vi "test wydajnosci akzwizycji.vi"() -> ()   [LabVIEW 2014]
uses:
  Kontrolki/KartaDAQ/ACQ analog channel config new.ctl
  Kontrolki/KartaDAQ/ACQ counter channel config.ctl
  Kontrolki/KartaDAQ/ACQ Params.ctl
  Kontrolki/KartaDAQ/ACQ all read tasks.ctl
  Kontrolki/FVGs/FVG akcje podstawowa.ctl
panel:
  out "srednie przysp":dbl
  out "srednia predk":dbl
  in  "generuj plik":bool
  in  "file path":path
  in  "Tab Control":enum32{"Page 1", "Page 2"}(tab)
  out "Waveform Graph":waveform(dbl)[](graph)
  out "Waveform Graph 3":waveform(dbl)[](graph)
  out "deleted portion":dbl[](array[numeric]) format="%.8f"
  out "Array":T1(array[cluster])
  out "size(s)":i32
  out "wektor size(s)":i32
  in  "użyj x0":bool
  out "okno dt":dbl
  out "dt":dbl
  out "średnia delay":dbl
  out "delay":dbl format="%.2f"
  in  "stop":bool
  in  "Urządzenie":tag="Dev1"
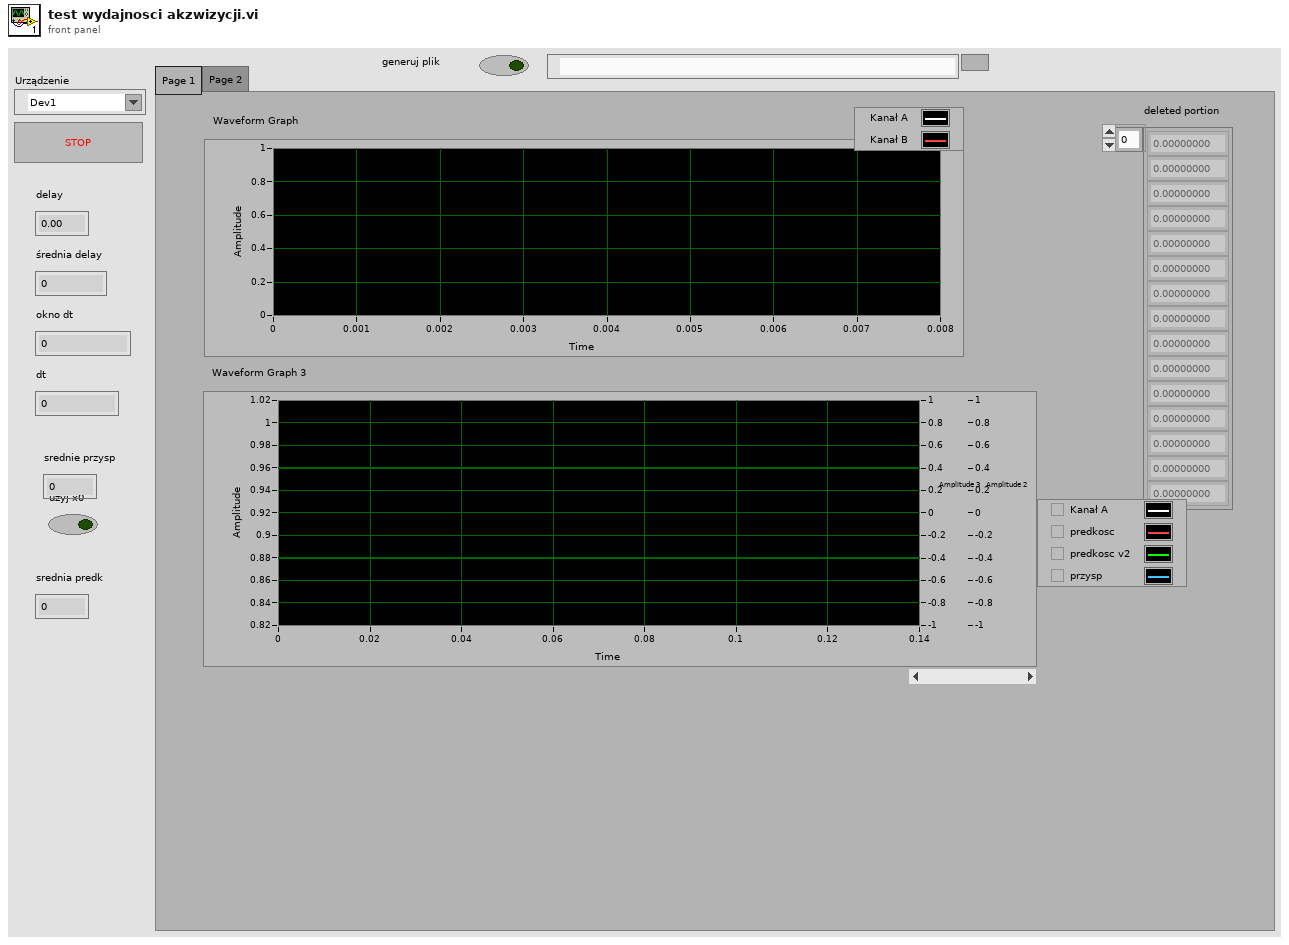
[diagram p1: front panel]
types:
  T1 = cluster{"dane":dbl[], "wygladzone":dbl[], "pochodna":dbl[], "pochodna wygl":dbl[]}[]
  T2 = typedef "ACQ all read tasks.ctl" = cluster{"Analog ref":refnum<k21>, "Enkoder X ref":refnum<k21>, "Enkoder Y ref":refnum<k21>, "Generator ref":refnum<k21>}
  T3 = typedef "ACQ Params.ctl" = cluster{"Analog":cluster{"minimum value":dbl, "maximum value":dbl}, "Digital":cluster{"minimum value":dbl, "maximum value":dbl}, "Time":cluster{"sample mode":i32, "samples per channel in":i32, "rate":dbl, "active edge":i32}, "AI common":cluster{"input terminal configuration":i32, "source":string}, "Enkoder":cluster{"channel1 name":string, "channel2 name":string, "units":i32, "initial position":dbl, "distance per pulse":dbl, "z index enable":bool, "z index value":dbl, "z index phase":i32, "decoding type":i32}}
  T4 = typedef "ACQ counter channel config.ctl" = cluster{"Enkoder X":string, "Enkoder Y":string, "Generator":string, "Generator OUT":string}
  T5 = typedef "ACQ analog channel config new.ctl" = cluster{"Analogs IN":string[], "Digitals IN":string[]}
  T6 = cluster{"dane":dbl[], "wygladzone":dbl[], "pochodna":dbl[], "pochodna wygl":dbl[]}
  T7 = typedef "FVG akcje podstawowa.ctl" = enum16{"GET", "SET"}
  T8 = enum16{"open", "open or create", "create or replace", "create", "open (read-only)"}
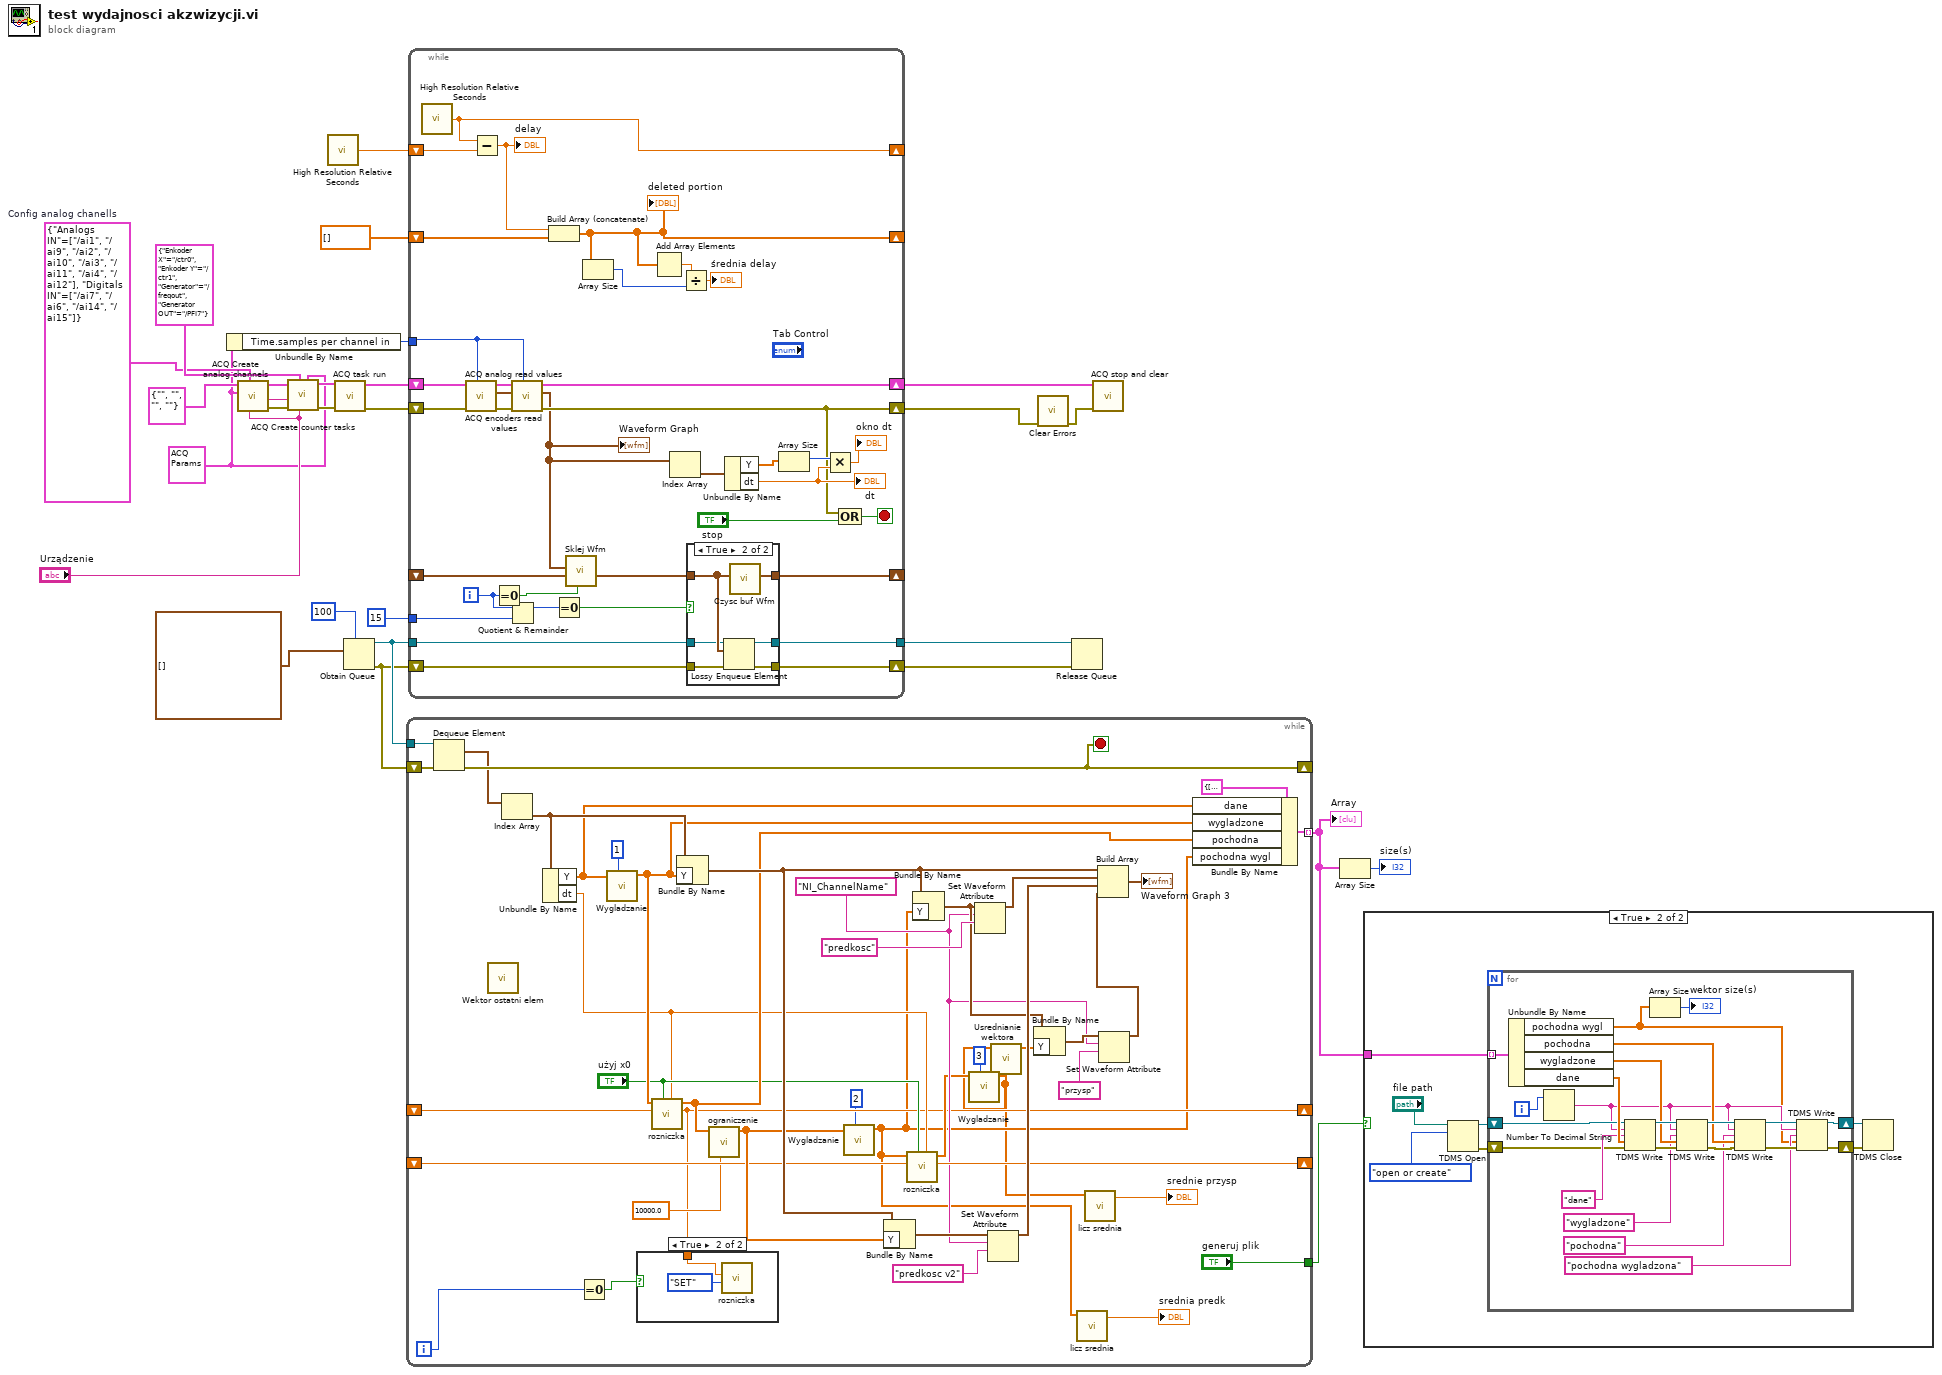
[diagram p0: block diagram]
diagram:
  w11 = T3 {"Analog"={"minimum value"=-1.0, "maximum value"=1.0}, "Digital"={"minimum value"=0.0, "maximum value"=5.0}, "Time"={"sample mode"=10123, "samples per channel in"=26, "rate"=3200.0, "active edge"=10280}, "AI common"={"input terminal configuration"=10083, "source"="/ai/SampleClock"}, "Enkoder"={"channel1 name"="Linear X", "channel2 name"="Linear Y", "units"=10219, "initial position"=0.0, "distance per pulse"=1.0, "z index enable"=FALSE, "z index value"=0.0, "z index phase"=10040, "decoding type"=10091}} ("ACQ Params")
  w19 = T5 {"Analogs IN"=["/ai1", "/ai9", "/ai2", "/ai10", "/ai3", "/ai11", "/ai4", "/ai12"], "Digitals IN"=["/ai7", "/ai6", "/ai14", "/ai15"]}  # Config analog chanells
  n1 = Unbundle By Name(w11) -> ("Time.samples per channel in"=w12:i32)
  n2 = call "ACQ Create analog channels.vi"("device in"="Urządzenie", "Config analog chanells new"=w19, "ACQ Params"=w11, "All Read tasks in"=T2 {"Analog ref"="", "Enkoder X ref"="", "Enkoder Y ref"="", "Generator ref"=""}) -> ("error out"=w15:errorcluster, "Terminal Name with Device Prefix"=w16:tag, "All Read tasks out"=w14:T2)  [unwired: 4 in, 1 out]
  n3 = call "ACQ Create counter tasks.vi"("ACQ Params"=w11, "device in"="Urządzenie", "Config Counter channels"=T4 {"Enkoder X"="/ctr0", "Enkoder Y"="/ctr1", "Generator"="/freqout", "Generator OUT"="/PFI7"}, "error in (no error)"=w15, "Terminal Name with Device Prefix"=w16, "All Read tasks in"=w14) -> ("error out"=w17:errorcluster, "All Read tasks out"=w18:T2)  [unwired: 4 in]
  n4 = call <vilib>:"High Resolution Relative Seconds.vi"() -> ("relative seconds"=w20:dbl)
  n5 = call "ACQ task run.vi"("error in (no error)"=w17, "All Read tasks in"=w18) -> ("error out"=w25:errorcluster, "All Read tasks out"=w26:T2)  [unwired: 7 in, 1 out]
  n6 = Obtain Queue(max queue size (-1, unlimited)=100, element data type=waveform(dbl)[] [] ("data")) -> (queue out=w7:refnum<queue>, error out=w4:errorcluster)  [unwired: 3 in, 1 out]
  n7 = while {
    tunnel: w7 -> [w70]
    shift-right: [w68] -> _
    shift-left: w4 -> [w69]
    shift-right: [w37] -> _
    shift-left: _ -> [w59]
    tunnel: [w55] -> w2 mode=indexing
    shift-right: [w51] -> _
    shift-left: _ -> [w50]
    tunnel: ["generuj plik"] -> w3
    i -> [w39]
    stop <- w68 stop-if-true
    w44 = "NI_ChannelName" ("name")
    n8 = Dequeue Element(queue=w70, error in (no error)=w69) -> (element=w67:waveform(dbl)[], error out=w68:errorcluster)  [unwired: 1 in, 2 out]
    n9 = call "Wektor ostatni elem.vi"() -> ()  [unwired: 11 in, 1 out]
    n10 = Index Array(array=w67) -> (element=w66:waveform(dbl))  [unwired: 1 in]
    n11 = Unbundle By Name(w66) -> ("Y"=w54:dbl[], "dt"=w41:dbl)
    n12 = Equal To 0?(x=w39) -> (x = 0?=w38:bool)
    n13 = call "Wygladzanie.vi"("Num (0..3)"=1, "Array in"=w54) -> ("Array out"=w53:dbl[])  [unwired: 9 in]
    n14 = call "rozniczka.vi"("dT"=w41, "użyj x0 (T)"="użyj x0", "x0"=w59, "Array in"=w53) -> ("ostatni"=w37:dbl, "Array out"=w56:dbl[])  [unwired: 6 in]
    n15 = case shown="True" w38 {
      tunnel: w37 -> [_ w71]
      frame False {
      }
      frame True {
        n16 = call "rozniczka.vi"("Akcja (GET)"=FVG_akcje_podstawowa."SET", "x0"=w71) -> ()  [unwired: 8 in, 2 out]
      }
    }
    n17 = Bundle By Name(cluster=w66, "Y"=w53) -> (w63:waveform(dbl))
    n18 = call "ograniczenie.vi"("dokladnosc"=10000.0, "Array in"=w56) -> ("Array"=w58:dbl[])  [unwired: 9 in]
    n19 = call "Wygladzanie.vi"("Num (0..3)"=2, "Array in"=w58) -> ("Array out"=w33:dbl[])  [unwired: 9 in]
    n20 = Bundle By Name(cluster=w63, "Y"=w58) -> (w62:waveform(dbl))
    n21 = call "rozniczka.vi"("dT"=w41, "użyj x0 (T)"="użyj x0", "x0"=w50, "Array in"=w33) -> ("ostatni"=w51:dbl, "Array out"=w42:dbl[])  [unwired: 6 in]
    n22 = Bundle By Name(cluster=w63, "Y"=w33) -> (w49:waveform(dbl))
    n23 = call "Wygladzanie.vi"("Num (0..3)"=3, "Array in"=w42) -> ("Array out"=w29:dbl[])  [unwired: 9 in]
    n24 = Set Waveform Attribute(5:"predkosc" ("name"), 6:w44, 7:w49) -> (3:w52:waveform(dbl))  [unwired: 1 in, 2 out]
    n25 = Set Waveform Attribute(5:"predkosc v2" ("name"), 6:w44, 7:w62) -> (3:w61:waveform(dbl))  [unwired: 1 in, 2 out]
    n26 = call "Usrednianie wektora.vi"("Array in"=w29) -> ("Array out"=w30:dbl[])  [unwired: 10 in]
    n27 = Bundle By Name(cluster=w49, "Y"=w30) -> (w46:waveform(dbl))
    n28 = call "licz srednia.vi"("Array in"=w33) -> ("Srednia"=→"srednia predk":dbl)  [unwired: 10 in]
    n29 = call "licz srednia.vi"("Array in"=w29) -> ("Srednia"=→"srednie przysp":dbl)  [unwired: 10 in]
    n30 = Set Waveform Attribute(5:"przysp" ("name"), 6:w44, 7:w46) -> (3:w45:waveform(dbl))  [unwired: 1 in, 2 out]
    n31 = Build Array(w63, w52, w61, w45) -> (→"Waveform Graph 3":waveform(dbl)[])
    n32 = Bundle By Name(cluster=T6 {"dane"=[], "wygladzone"=[], "pochodna"=[], "pochodna wygl"=[]} ("Cluster"), "dane"=w54, "wygladzone"=w53, "pochodna"=w56, "pochodna wygl"=w33) -> (w55:T6)
  }
  "Array" <- w2
  n33 = while {
    shift-right: [w88] -> w23
    shift-left: w26 -> [w108]
    shift-right: [w87] -> w22
    shift-left: w25 -> [w107]
    shift-right: [w92] -> _
    shift-left: w20 -> [w106]
    shift-right: [w94] -> _
    shift-left: dbl[] [] -> [w105]
    tunnel: w12 -> [w86]
    tunnel: 15 ("y") -> [w80]
    shift-right: [w82] -> _
    shift-left: _ -> [w84]
    tunnel: w7 -> [w76]
    tunnel: [w74] -> w6
    shift-right: [w73] -> w5
    shift-left: w4 -> [w75]
    i -> [w79]
    stop <- w96 stop-if-true
    n34 = call <vilib>:"High Resolution Relative Seconds.vi"() -> ("relative seconds"=w92:dbl)
    n35 = call "ACQ analog read values.vi"("samples per channel"=w86, "error in (no error)"=w107, "Tasks ref in"=w108) -> ("error out"=w89:errorcluster, "data"=w90:waveform(dbl)[], "Tasks ref out"=w91:T2)  [unwired: 6 in]
    n36 = Subtract(x=w92, y=w106) -> (x-y=w97:dbl)
    "delay" <- w97
    n37 = Equal To 0?(x=w79) -> (x = 0?=w78:bool)
    n38 = Quotient & Remainder(x=w79, y=w80) -> (x-y*floor(x/y)=w81:i32)  [unwired: 1 out]
    n39 = call "ACQ encoders read values.vi"("samples per channel"=w86, "error in (no error)"=w89, "AI data"=w90, "Tasks ref in"=w91) -> ("error out"=w87:errorcluster, "Enk wfm out"=w85:waveform(dbl)[], "Tasks ref out"=w88:T2)  [unwired: 5 in]
    "Waveform Graph" <- w85
    n40 = Build Array (concatenate)(w97, w105) -> (w94:dbl[])
    "deleted portion" <- w94
    n41 = Equal To 0?(x=w81) -> (x = 0?=w77:bool)
    n42 = call "Sklej Wfm.vi"("zerowy?"=w78, "Wfm Bufor in"=w84, "Wfm New data"=w85) -> ("Wfm Bufor out"=w83:waveform(dbl)[])  [unwired: 7 in, 1 out]
    n43 = Array Size(array=w94) -> (size(s)=w93:i32)
    n44 = Add Array Elements(numeric array=w94) -> (sum=w104:dbl)
    n45 = Index Array(array=w85) -> (element=w102:waveform(dbl))  [unwired: 1 in]
    n46 = Divide(x=w104, y=w93) -> (x/y=→"średnia delay":dbl)
    n47 = case shown="True" w77 {
      tunnel: w83 -> [w111 w116]
      tunnel: [w111 w117] -> w82
      tunnel: w76 -> [w110 w115]
      tunnel: w75 -> [w109 w114]
      tunnel: [w110 w113] -> w74
      tunnel: [w109 w112] -> w73
      frame False {
      }
      frame True {
        n48 = Lossy Enqueue Element(queue=w115, element=w116, error in (no error)=w114) -> (queue out=w113:refnum<queue>, error out=w112:errorcluster)  [unwired: 2 out]
        n49 = call "Czysc buf Wfm.vi"("Wfm Bufor in"=w116) -> ("Wfm Bufor out"=w117:waveform(dbl)[])  [unwired: 10 in]
      }
    }
    n50 = Unbundle By Name(w102) -> ("Y"=w101:dbl[], "dt"=w100:dbl)
    "dt" <- w100
    n51 = Array Size(array=w101) -> (size(s)=w99:i32)
    n52 = Multiply(x=w99, y=w100) -> (x*y=→"okno dt":dbl)
    n53 = Compound Arithmetic op=OR(w87, "stop") -> (w96:bool)
  }
  n54 = call <vilib>:"Clear Errors.vi"("error in (no error)"=w22) -> ("error out"=w24:errorcluster)  [unwired: 5 in, 1 out]
  n55 = Release Queue(queue=w6, error in (no error)=w5) -> ()  [unwired: 1 in, 3 out]
  n56 = call "ACQ stop and clear.vi"("error in (no error)"=w24, "Tasks ref in"=w23) -> ()  [unwired: 9 in, 1 out]
  n57 = Array Size(array=w2) -> (size(s)=→"size(s)":i32)
  n58 = case shown="True" w3 {
    tunnel: w2 -> [_ w120]
    frame False {
    }
    frame True {
      n59 = TDMS Open(10:T8."open or create" ("operation (0:open)"), 11:"file path") -> (0:w123:errorcluster, 3:w124:refnum<k34>)  [unwired: 5 in]
      n60 = for {
        shift-right: [w138] -> w121
        shift-left: w124 -> [w130]
        shift-right: [w139] -> w122
        shift-left: w123 -> [w129]
        tunnel: w120 -> [w146] mode=indexing
        i -> [w128]
        n61 = Unbundle By Name(w146) -> ("pochodna wygl"=w125:dbl[], "pochodna"=w135:dbl[], "wygladzone"=w136:dbl[], "dane"=w137:dbl[])
        n62 = Number To Decimal String(number=w128) -> (decimal integer string=w127:string)  [unwired: 1 in]
        n63 = TDMS Write(0:w130, 5:w127, 7:"dane", 9:w137, 11:w129) -> (4:w145:refnum<k34>, 15:w144:errorcluster)  [unwired: 1 in, 2 out]
        n64 = Array Size(array=w125) -> (size(s)=→"wektor size(s)":i32)
        n65 = TDMS Write(0:w145, 5:w127, 7:"wygladzone", 9:w136, 11:w144) -> (4:w142:refnum<k34>, 15:w143:errorcluster)  [unwired: 1 in, 2 out]
        n66 = TDMS Write(0:w142, 5:w127, 7:"pochodna", 9:w135, 11:w143) -> (4:w140:refnum<k34>, 15:w141:errorcluster)  [unwired: 1 in, 2 out]
        n67 = TDMS Write(0:w140, 5:w127, 7:"pochodna wygladzona", 9:w125, 11:w141) -> (4:w138:refnum<k34>, 15:w139:errorcluster)  [unwired: 1 in, 2 out]
      }
      n68 = TDMS Close(8:w122, 11:w121) -> ()  [unwired: 2 out]
    }
  }
